vi "ParseJsonStringForData.vi"() -> ()   [LabVIEW 2020]
uses:
  <vilib>/NI/JSON Support for LabVIEW/JSON Value/JSON Value.lvclass
panel:
  out "Array":string[][](array[string])
  in  "JSON String":string
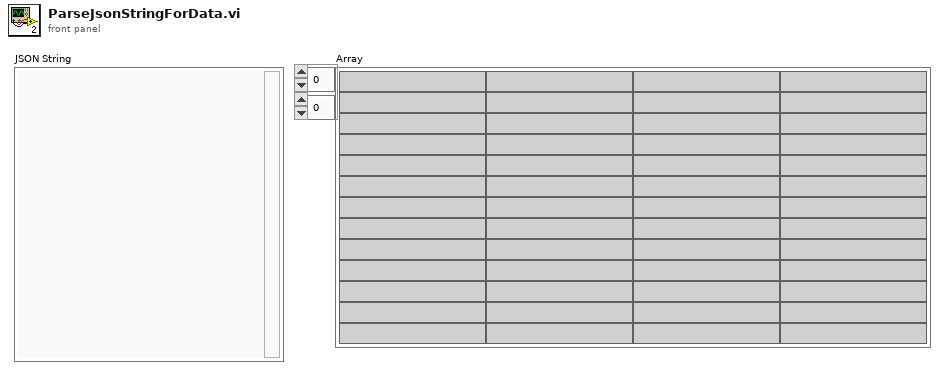
[diagram p1: front panel]
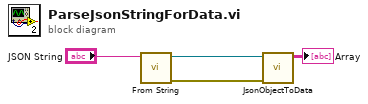
[diagram p0: block diagram]
diagram:
  n1 = call <vilib>:"From String.vi"("JSON String"="JSON String") -> ("error out"=w2:errorcluster, "JSON Value out"=w3:refnum<class "JSON Value.lvclass">)  [unwired: 9 in]
  n2 = call "JsonObjectToData.vi"("error in (no error)"=w2, "JSON Value in"=w3) -> ("Array"=→"Array":string[][])  [unwired: 9 in]
